vi "test_DDS_generator.vi"() -> ()   [LabVIEW 2018]
panel:
  out "Waveform Graph":dbl[](graph)
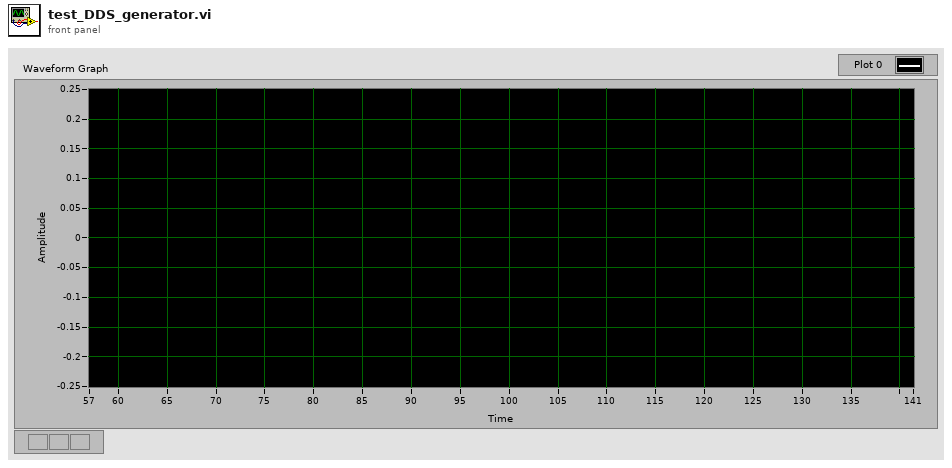
[diagram p1: front panel]
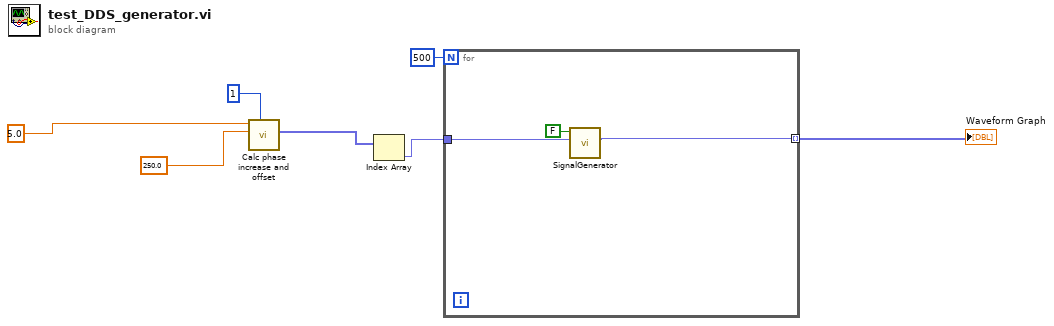
[diagram p0: block diagram]
diagram:
  n1 = call "Calc phase increase and offset.vi"("# of DDS"=1, "fclk (MHz)"=250.0 ("fclk (800MHz)"), "f_generated (MHz)"=5.0 ("Output mixer fequency [MHz]")) -> ("Phase out"=w2:fxp<+,64,64>[])  [unwired: 6 in, 2 out]
  n2 = Index Array(array=w2) -> (element=w1:fxp<+,64,64>)  [unwired: 1 in]
  n3 = for {
    N: 500 -> [_]
    tunnel: [w10] -> w3 mode=indexing
    tunnel: w1 -> [w9]
    n4 = call "SignalGenerator.vi"("phase"=w9, "Reset"=FALSE) -> ("Sin"=w10:fxp<+/-,16,0>)  [unwired: 7 in, 2 out]
  }
  "Waveform Graph" <- w3
